vi "Data Source Exitport.vi"() -> (1 "Add?":bool, 2 "OK?":bool, 3 "Data":string[][](array[string]))   [LabVIEW 2020]
uses:
  <vilib>/Utility/NIReport.llb/NI_report.lvclass
  <vilib>/Utility/NIReport.llb/Excel/NI_Excel.lvclass
  <vilib>/Utility/NIReport.llb/Report Type.ctl
  <vilib>/Utility/NIReport.llb/NI_ReportGenerationCore.lvlib
  <vilib>/addons/_office/NI_ReportGenerationToolkit.lvlib
  <vilib>/Utility/miscctls.llb/LVRowAndColumnUnsignedTypeDef.ctl
  <vilib>/addons/_office/excel.llb/Excel Get Data ([str]).vi
panel:
  in  "Data Source":i32(listbox)
  in  "Cancle":bool
  in  "Cover":bool
  in  "Add":bool
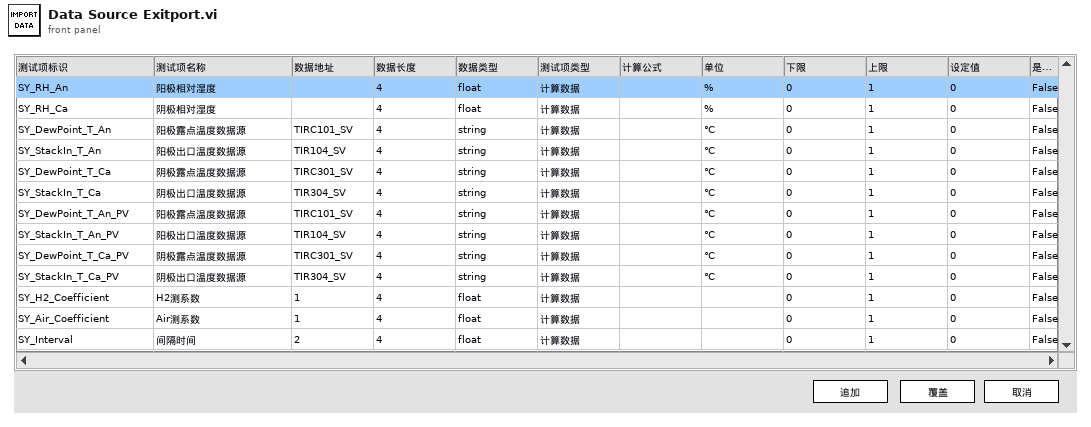
[diagram p1: front panel]
types:
  T1 = enum32{"Invalid", "Standard", "Closed", "Hidden", "Minimized", "Maximized"}
  T2 = typedef "LVRowAndColumnUnsignedTypeDef.ctl" = cluster{"Row":u32, "Column":u32}
  T3 = enum16{"maximized", "minimized", "normal", "no change"}
  T4 = typedef "NI_ReportGenerationCore.lvlib/Report Type.ctl" = enum16{"HTML", "Word", "Excel"}
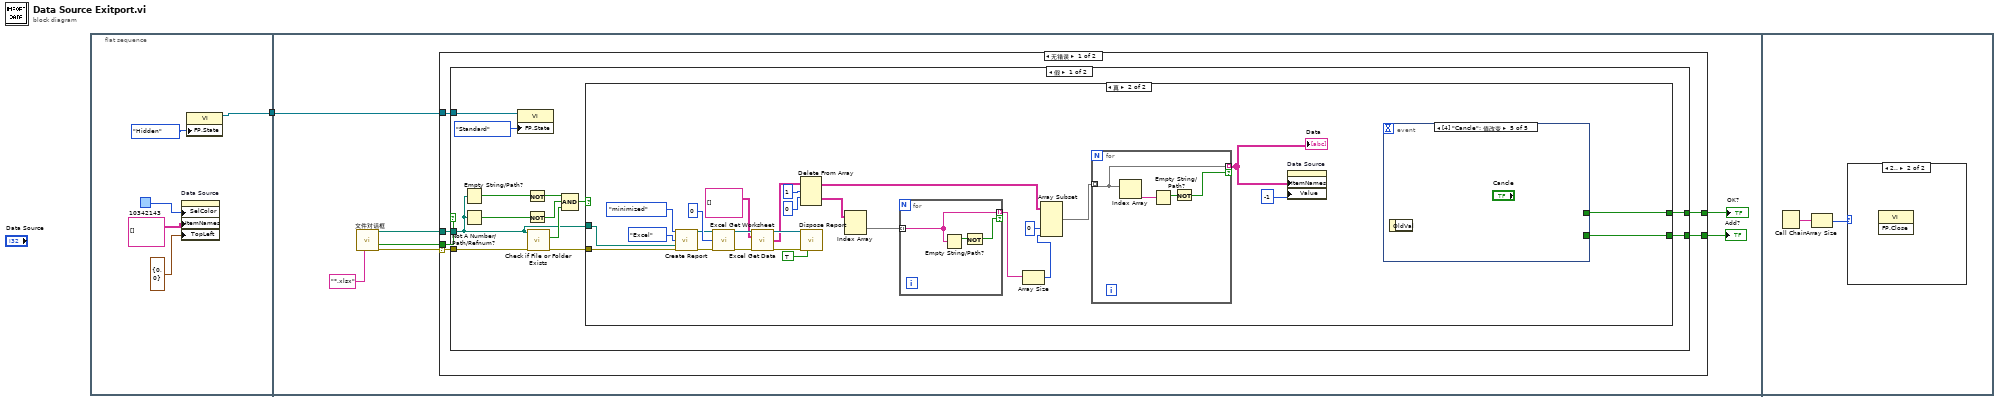
[diagram p0: block diagram]
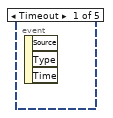
[diagram p3: hidden frame]
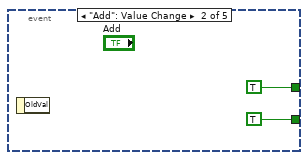
[diagram p4: hidden frame]
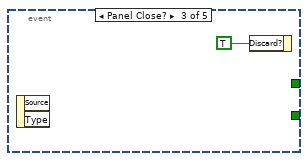
[diagram p5: hidden frame]
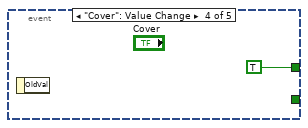
[diagram p6: hidden frame]
diagram:
  n1 = flat-sequence {
    tunnel: [w2] -> w1
    tunnel: w1 -> [w7]
    frame #0 {
      n2 = property on="Data Source" class="MCListbox (严格)"("SelColor"=u32 10342143 ("选择颜色"), "ItemNames"=string[][] [] ("项名"), "TopLeft"=T2 {"Row"=0, "Column"=0} ("左上可见单元格")) -> ()  [unwired: 2 in, 2 out]
      n3 = property class="VI"("FP.State"=T1."Hidden" ("前面板窗口:状态")) -> (reference out=w2:refnum<vi>)  [unwired: 2 in, 1 out]
    }
    frame #1 {
      n4 = call "文件对话框"("pattern (all files)"="*.xlsx") -> ("selected path"=w10:path, "cancelled"=w12:bool, "error out"=w11:errorcluster)  [unwired: 11 in, 1 out]
      n5 = case shown="无错误" w11 {
        selector: w11 -> [w17 _]
        tunnel: w12 -> [w19 _]
        tunnel: w10 -> [w18 _]
        tunnel: [w16 _] -> w9
        tunnel: [w15 _] -> w8
        tunnel: w7 -> [w14 _]
        frame No Error {
          n6 = case shown="假" w19 {
            tunnel: w18 -> [w27 _]
            tunnel: w17 -> [w25 _]
            tunnel: [w23 _] -> w16
            tunnel: [w22 _] -> w15
            tunnel: w14 -> [w21 _]
            frame False {
              n7 = Empty String/Path?(string/path=w27) -> (empty?=w32:bool)
              n8 = Not A Number/Path/Refnum?(number/path/refnum=w27) -> (NaN/Path/Refnum?=w31:bool)
              n9 = property class="VI"(reference=w21, "FP.State"=T1."Standard" ("前面板窗口:状态")) -> ()  [unwired: 1 in, 2 out]
              n10 = Not(x=w32) -> (.not. x?=w30:bool)
              n11 = Not(x=w31) -> (.not. x?=w29:bool)
              n12 = call <vilib>:"Check if File or Folder Exists.vi"("error in (no error)"=w25, "path"=w27) -> ("error out"=w24:errorcluster, "file or folder exists?"=w28:bool)  [unwired: 7 in, 1 out]
              n13 = Compound Arithmetic op=AND ("复合运算")(w30, w29, w28) -> (w26:bool)
              n14 = case shown="真" w26 {
                tunnel: w27 -> [_ w45]
                tunnel: w24 -> [_ w44]
                tunnel: [_ w42] -> w23
                tunnel: [_ w41] -> w22
                frame False {
                }
                frame True {
                  n15 = call <vilib>:"Create Report.vi"("window state (normal)"=T3."minimized", "report type"=Report_Type."Excel", "template (empty)"=w45, "error in (no error)"=w44) -> ("report out"=w58:refnum<class "NI_report.lvclass">, "error out"=w57:errorcluster)  [unwired: 10 in]
                  n16 = call <vilib>:"Excel Get Worksheet.vi"("report in"=w58, "worksheet index (0)"=0, "error in (no error)"=w57) -> ("report out"=w54:refnum<class "NI_report.lvclass">, "error out"=w55:errorcluster)  [unwired: 11 in]
                  n17 = call-poly <vilib>:"Excel Get Data.vi"("report in"=w54, "data type"=string[][] [], "error in (no error)"=w55) -> ("report out"=w51:refnum<class "NI_report.lvclass">, "data"=w48:string[][], "error out"=w52:errorcluster)  [unwired: 10 in]
                  n18 = Delete From Array(array=w48, length=1 ("长度"), index (row)=0 ("索引 (行)")) -> (deleted portion=w34:string[][], array with subset deleted=w39:string[][])  [unwired: 1 in]
                  n19 = call-dynamic "Dispose Report.vi"("report in"=w51, "error in (no error)"=w52, "close report? (T)"=TRUE) -> ()  [unwired: 12 in, 1 out]
                  n20 = Index Array(array=w34) -> (element=w33:string[])  [unwired: 2 in]
                  n21 = for {
                    tunnel: [w60] -> w37 mode=indexing if=w61
                    tunnel: w33 -> [w60] mode=indexing
                    n22 = Empty String/Path?(string/path=w60) -> (empty?=w62:bool)
                    n23 = Not(x=w62) -> (.not. x?=w61:bool)
                  }
                  n24 = Array Size(array=w37) -> (size(s)=w36:i32)
                  n25 = Array Subset(array=w39, index (col)=0 ("索引"), length (col)=w36) -> (w35:string[][])  [unwired: 2 in]
                  n26 = for {
                    tunnel: w35 -> [w66] mode=indexing
                    tunnel: [w66] -> w40 mode=indexing if=w63
                    n27 = Index Array(array=w66) -> (element=w65:string)  [unwired: 1 in]
                    n28 = Empty String/Path?(string/path=w65) -> (empty?=w64:bool)
                    n29 = Not(x=w64) -> (.not. x?=w63:bool)
                  }
                  "Data" <- w40
                  n30 = property on="Data Source" class="MCListbox (严格)"("ItemNames"=w40, "Value"=-1 ("Data Source")) -> ()  [unwired: 2 in, 2 out]
                  n31 = event shown="[4] \"Cancle\": 值改变" {
                    selector: _ -> [_ _ _ _ _]
                    dyn-events: _ -> [_ _ _ _ _]
                    timeout: _ -> [_ _ _ _ _]
                    tunnel: [_ TRUE _ TRUE _] -> w42
                    tunnel: [_ TRUE _ _ _] -> w41
                    event Timeout {
                      n32 = event-data() -> ()  [unwired: 1 in, 3 out]
                    }
                    event "Add": Value Change {
                      n33 = event-data() -> ()  [unwired: 1 in, 1 out]
                    }
                    event Panel Close? {
                      n34 = event-data() -> ()  [unwired: 1 in, 2 out]
                      n35 = event-data("Discard?"=TRUE ("放弃？")) -> ()  [unwired: 1 in, 1 out]
                    }
                    event "Cover": Value Change {
                      n36 = event-data() -> ()  [unwired: 1 in, 1 out]
                    }
                    event "Cancle": Value Change {
                      n37 = event-data() -> ()  [unwired: 1 in, 1 out]
                    }
                  }
                }
              }
            }
            frame True {
            }
          }
        }
        frame Error {
        }
      }
      "OK?" <- w9
      "Add?" <- w8
    }
    frame #2 {
      n38 = Call Chain() -> (call chain=w72:string[])
      n39 = Array Size(array=w72) -> (size(s)=w71:i32)
      n40 = case shown="2.." w71 {
        frame 0, Default {
        }
        frame 2.. {
          n41 = invoke class="VI" method="FP.Close"() -> ()  [unwired: 3 in, 3 out]
        }
      }
    }
  }
